vi "Test State Data Size Correct.vi"(8 "error in (no error)":errorcluster, 11 "Test Case In":refnum<class "Debugger Test.lvclass">) -> (0 "error out":errorcluster, 3 "Test Case Out":refnum<class "Debugger Test.lvclass">)   [LabVIEW 2020, in "Debugger Test.lvclass"]
uses:
  Debugger Test.lvclass
  C:/Program Files (x86)/National Instruments/LabVIEW 2020/vi.lib/Astemes/LUnit/Test Case.lvclass
  source/Debugger/Debugger.lvclass
  C:/Users/anton/Documents/GitHub/triarc-debugger/source/Process/Debug Process.lvclass
  source/Debug Data/Raw Debug Data.ctl
  source/Process/Debug Process.lvclass/Debug Process.ctl
  source/Debug Data/Debug Data.lvclass/Debug Data.ctl
  <vilib>/Astemes/LUnit/Test Case.lvclass/Test Case.ctl
  <vilib>/Astemes/LUnit/LUnit Assertion Result.lvclass/LUnit Assertion Result.ctl
  <vilib>/Astemes/LUnit/LUnit Test Case Result.lvclass/LUnit Test Case Result.ctl
  <vilib>/Astemes/LUnit/LUnit Method Result.lvclass/LUnit Method Result.ctl
  01074fa8-ee8a-411d-bc8b-fc92c4f90959.vi
  source/Process/Public/Lifecycle/Get Lifecycle State.vi
  <vilib>/AdvancedString/Delimited String to 1D String Array.vi
  <vilib>/Astemes/Triarc Framework/Broadcast Event Helpers/Execution timer.vi
  source/Process/Private/SubVIs/Wait for finish.vi
  source/Process/Protected/Messaging/Enqueue Message.vi
  source/Process/Private/SubVIs/Set Lifecycle State.vi
  <vilib>/Astemes/LUnit/Palette/Pass.vi
  <vilib>/Astemes/LUnit/Palette/Fail.vi
  <vilib>/Astemes/LUnit/Compare Variants.vi
  <vilib>/Astemes/LUnit/Describe Comparison.vi
  <vilib>/Astemes/LUnit/Set Assertion Type.vi
  <vilib>/Utility/error.llb/Clear Errors.vi
  <vilib>/Astemes/LUnit/Add test result.vi
  <vilib>/Astemes/LUnit/LUnit Write Passed.vi
  <vilib>/Astemes/LUnit/LUnit Write Message.vi
  <vilib>/Astemes/LUnit/LUnit Write Description.vi
  <vilib>/Astemes/LUnit/Variant to string.vi
  <vilib>/Astemes/LUnit/LUnit Write Assertion Type.vi
  <vilib>/Astemes/LUnit/LUnit Record Assertion Result.vi
  <vilib>/Astemes/LUnit/LUnit Aggregate Assertion Results.vi
  <vilib>/Astemes/LUnit/Assertion Result/LUnit Read Status.vi
  <vilib>/Astemes/LUnit/LUnit Read Message.vi
  <vilib>/Astemes/LUnit/LUnit Read Description.vi
  <vilib>/Astemes/LUnit/Method Result/LUnit Merge Status.vi
  <vilib>/Astemes/LUnit/LUnit Concatenate result strings.vi
  <vilib>/Utility/error.llb/Error Cluster From Error Code.vi
  <vilib>/Astemes/Triarc Framework/Broadcast Event Helpers/Dequeue Broadcast Message.vi
  <vilib>/Utility/Data Type/Get Type Information.vi
  <vilib>/Utility/LVClass/Get LV Class Name.vi
  source/Debug Data/Debug Data.lvclass
  <vilib>/Astemes/LUnit/LUnit Assertion Result.lvclass
  source/Process/Debug Process.lvclass
  <vilib>/Astemes/Triarc Framework/Broadcast Event Helpers/Broadcast Event Helpers.lvlib
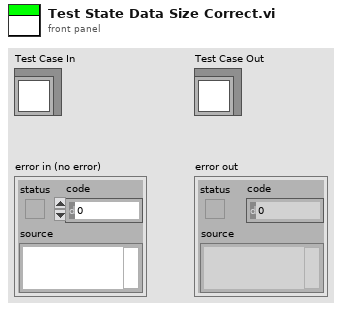
[diagram p1: front panel]
types:
  T1 = typedef "Debug Data.lvclass/Raw Debug Data.ctl" = cluster{"Action":string, "Call Chain":string, "Process":string, "Message":string, "Message Data":variant, "Time":dbl}
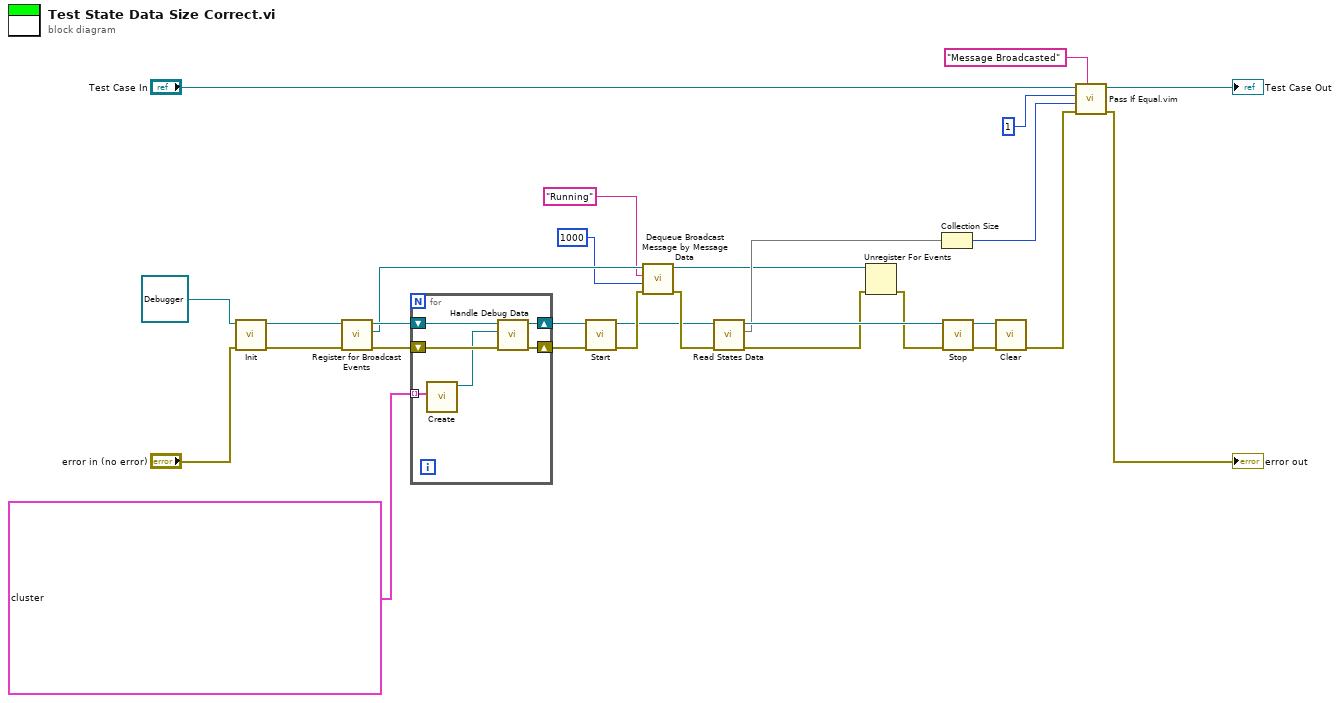
[diagram p0: block diagram]
diagram:
  n1 = call-dynamic "Init.vi"("error in (no error)"="error in (no error)", "Process In"=refnum<class "Debugger.lvclass"> refnum ("Debug Data Event In 2")) -> ("error out"=w3:errorcluster, "Process Out"=w4:refnum<class "Debugger.lvclass">)  [unwired: 8 in]
  n2 = call "Register for Broadcast Events.vi"("error in (no error)"=w3, "Process In"=w4) -> ("error out"=w26:errorcluster, "Event Registration Refnum Out"=w17:refnum<event-registration>, "Process Out"=w22:refnum<class "Debugger.lvclass">)  [unwired: 7 in]
  n3 = for {
    shift-right: [w33] -> w9
    shift-left: w26 -> [w35]
    shift-right: [w34] -> w6
    shift-left: w22 -> [w32]
    tunnel: T1[] [{"Action"="Send", "Call Chain"="Test.vi:123456", "Process"="Process 1", "Message"="Init", "Message Data"=variant, "Time"=0.0}, {"Action"="Receive", "Call Chain"="TF.lvlib:Process.lvclass:Handle Messages.vi:1960001", "Process"="Process 1", "Message"="Init", "Message Data"=variant, "Time"=0.0}, {"Action"="Send", "Call Chain"="Test.vi", "Process"="Process 1", "Message"="Start", "Message Data"=variant, "Time"=0.0}, {"Action"="Receive", "Call Chain"="Test.vi", "Process"="Process 1", "Message"="Start", "Message Data"=variant, "Time"=0.0}] ("Debug Data Cluster") -> [w30] mode=indexing
    n4 = call "Create.vi"("Debug Data Cluster"=w30) -> ("Debug Data out"=w31:refnum<class "Debug Data.lvclass">)  [unwired: 9 in, 1 out]
    n5 = call-dynamic "Handle Debug Data.vi"("error in (no error)"=w35, "Debug Data.lvclass"=w31, "Debug Data Event In"=w32) -> ("error out"=w33:errorcluster, "Debug Data Event Out"=w34:refnum<class "Debugger.lvclass">)  [unwired: 7 in]
  }
  n6 = call "Start.vi"("error in (no error)"=w9, "Process In"=w6) -> ("error out"=w7:errorcluster, "Process Out"=w5:refnum<class "Debugger.lvclass">)  [unwired: 7 in, 1 out]
  n7 = call <vilib>:"Dequeue Broadcast Message by Message Data.vi"("error in (no error)"=w7, "Timeout (-1)"=1000, "Message Data"="Running", "Event Registration Refnum"=w17) -> ("error out"=w8:errorcluster, "Event Registration Refnum Out"=w10:refnum<event-registration>)  [unwired: 3 in, 3 out]
  n8 = call "Read States Data.vi"("error in (no error)"=w8, "Debugger in"=w5) -> ("error out"=w16:errorcluster, "State Map"=w11:map{string, string}, "Debugger in 2"=w25:refnum<class "Debugger.lvclass">)  [unwired: 7 in]
  n9 = Unregister For Events(event registration refnum=w10, error in=w16) -> (error out=w15:errorcluster)
  n10 = Collection Size(1:w11) -> (0:w13:i32)
  n11 = call "Stop.vi"("error in (no error)"=w15, "Process In"=w25) -> ("error out"=w23:errorcluster, "Process Out"=w24:refnum<class "Debugger.lvclass">)  [unwired: 7 in, 1 out]
  n12 = call-dynamic "Clear.vi"("error in (no error)"=w23, "Process In"=w24) -> ("error out"=w19:errorcluster)  [unwired: 9 in]
  n13 = call "Pass If Equal.vim"("Description"="Message Broadcasted", "error in (no error)"=w19, "Actual"=w13, "Expected"=1 ("size"), "LUnit Test Case In"="Test Case In") -> ("error out"=→"error out":errorcluster, "LUnit Test Case Out"=→"Test Case Out":refnum<class "Debugger Test.lvclass">)  [unwired: 5 in]
